vi "Delete Common FP Controls.vi"(8 "error in":errorcluster, 9 "Control FP Order":i32[](array[numeric]), 10 "Ref. VI":refnum<vi>) -> (0 "error out":errorcluster)   [LabVIEW 2025, in "_Msg Rescript.lvlib" / "_Msg Rescript.lvclass"]
uses:
  _Msg Rescript.lvclass
  _Msg Rescript.lvclass/_Msg Rescript.ctl
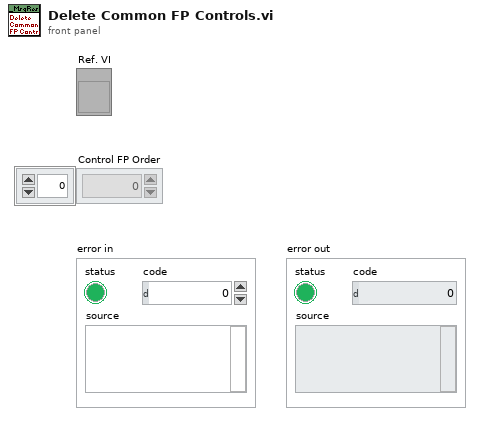
[diagram p1: front panel]
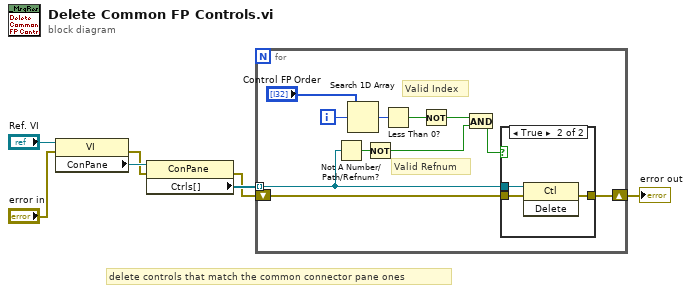
[diagram p0: block diagram]
diagram:
  # "delete controls that match the common connector pane ones"
  n1 = property class="VI"(reference="Ref. VI", error in="error in") -> (error out=w4:errorcluster, "ConPane"=w7:refnum<vi>)  [unwired: 1 out]
  n2 = property class="ConPane"(reference=w7, error in=w4) -> (error out=w5:errorcluster, "Ctrls[]"=w6:refnum<vi>[])  [unwired: 1 out]
  n3 = for {
    tunnel: w6 -> [w9] mode=indexing
    shift-right: [w16] -> w1
    shift-left: w5 -> [w15]
    i -> [w18]
    # "Valid Refnum"
    # "Valid Index"
    n4 = Not A Number/Path/Refnum?(number/path/refnum=w9) -> (NaN/Path/Refnum?=w13:bool)
    n5 = Search 1D Array(1D array="Control FP Order", element=w18) -> (index of element=w17:i32)  [unwired: 1 in]
    n6 = Not(x=w13) -> (.not. x?=w12:bool)
    n7 = Less Than 0?(x=w17) -> (x < 0?=w10:bool)
    n8 = Not(x=w10) -> (.not. x?=w11:bool)
    n9 = And(x=w11, y=w12) -> (x .and. y?=w8:bool)
    n10 = case shown="True" w8 {
      tunnel: w9 -> [_ w22]
      tunnel: [w19 w21] -> w16
      tunnel: w15 -> [w19 w20]
      frame False {
      }
      frame True {
        n11 = invoke class="Ctl" method="Delete"(reference=w22, error in=w20) -> (error out=w21:errorcluster)  [unwired: 1 in, 2 out]
      }
    }
  }
  "error out" <- w1
